vi "defendGoalTacticCheckStateChange.vi"(8 "error in (no error)":errorcluster, 11 "DefendGoalTacticVSS in":refnum<class "DefendGoalTacticVSS.lvclass">) -> (0 "error out":errorcluster, 2 "States":enum16{"Kick", "DefBallPos", "Exit"}(ring), 3 "DefendGoalTacticVSS out":refnum<class "DefendGoalTacticVSS.lvclass">)   [LabVIEW 2020, in "DefendGoalTacticVSS.lvclass"]
uses:
  DefendGoalTacticVSS.lvclass
  Robot_class/Robot.lvclass
  Game_class/Game.lvclass
  Utilities_class/Utilities.lvclass
  Game_class/Game.lvclass/Game.ctl
  Game_class/Read BallRef.vi
  Object_class/Read x.vi
  Ball_class/Ball.lvclass
panel:
  in  "Game in":refnum<class "Game.lvclass">
  in  "Robot":refnum<class "Robot.lvclass">
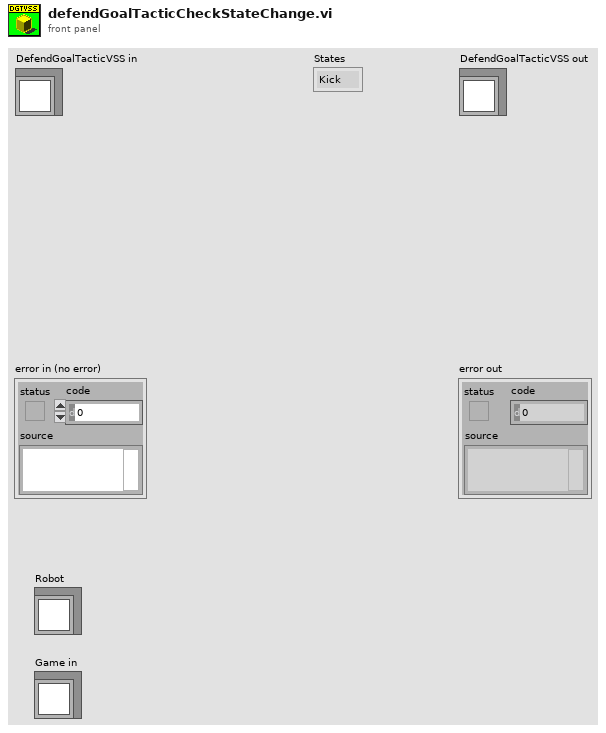
[diagram p1: front panel]
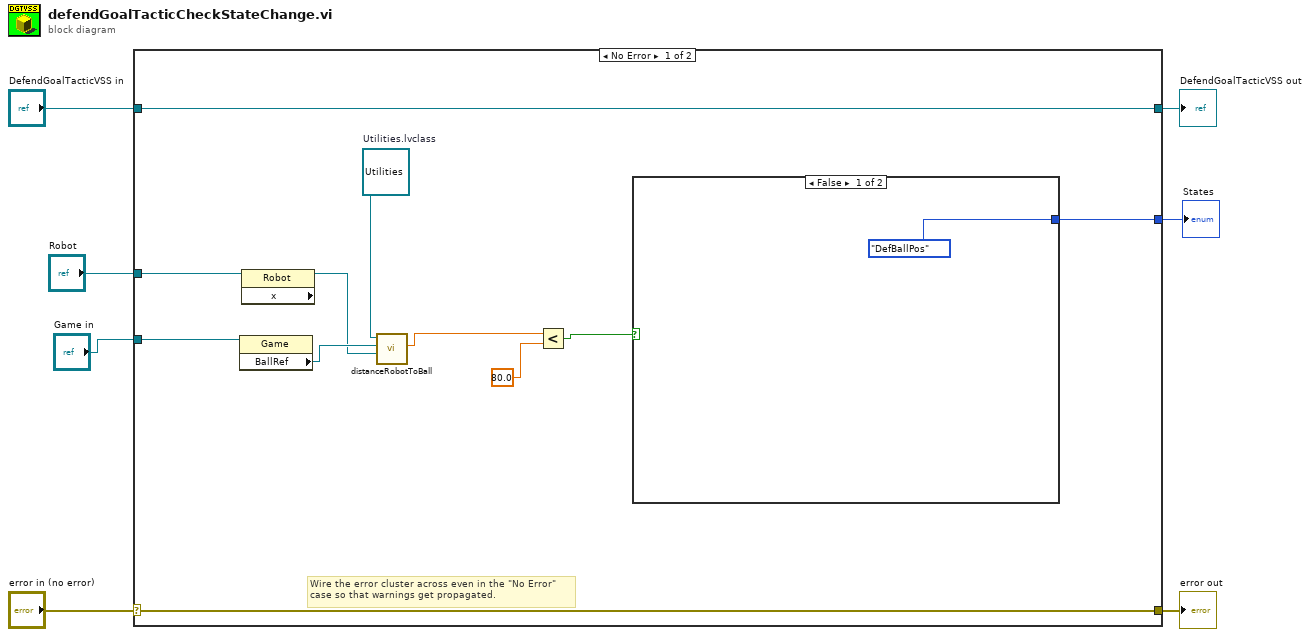
[diagram p0: block diagram]
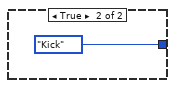
[diagram p2: hidden frame]
diagram:
  n1 = case shown="No Error" "error in (no error)" {
    selector: "error in (no error)" -> [w17 w22]
    tunnel: [w17 w22] -> w6
    tunnel: [w18 w21] -> w4
    tunnel: "DefendGoalTacticVSS in" -> [w18 w21]
    tunnel: [w16 _] -> w3
    tunnel: "Robot" -> [w15 _]
    tunnel: "Game in" -> [w14 _]
    frame No Error {
      w12 = refnum<class "Utilities.lvclass"> refnum  # Utilities.lvclass
      # "Wire the error cluster across even in the \"No Error\"\ncase so that warnings get propagated."
      n2 = property class="Game"(reference=w14) -> ("BallRef"=w11:refnum<class "Ball.lvclass">)  [unwired: 1 in, 2 out]
      n3 = property class="Robot" props=["x"](reference=w15) -> (reference out=w10:refnum<class "Robot.lvclass">)  [unwired: 1 in, 2 out]
      n4 = call "distanceRobotToBall.vi"("Robot"=w10, "Ball"=w11, "Utilities in"=w12) -> ("Distance Robot To Ball"=w9:dbl)  [unwired: 6 in, 2 out]
      n5 = Less?(x=w9, y=80.0) -> (x < y?=w8:bool)
      n6 = case shown="False" w8 {
        tunnel: [enum16{"Kick", "DefBallPos", "Exit"}."DefBallPos" enum16{"Kick", "DefBallPos", "Exit"}."Kick"] -> w16
        frame False {
        }
        frame True {
        }
      }
    }
    frame Error {
    }
  }
  "error out" <- w6
  "DefendGoalTacticVSS out" <- w4
  "States" <- w3
